vi "CSMinfo.vi"(4 "Error In":errorcluster, 7 "Command":string) -> (0 "Error Out":errorcluster, 3 "Response":string)   [LabVIEW 2018]
uses:
  MOKO_LabViewLibrary/MokoLowLevel/MokoLowLovelControl/MLLC_Mode.ctl
  data/CSMinfo.ctl
panel:
  in  "Utility name":string="CSMinfo"
  in  "Error Code":i32=5475
  in  "Settings":T2
  in  "Mode":T3=enum."Check"
  # "CSMinfo"
  # "Default Settings"
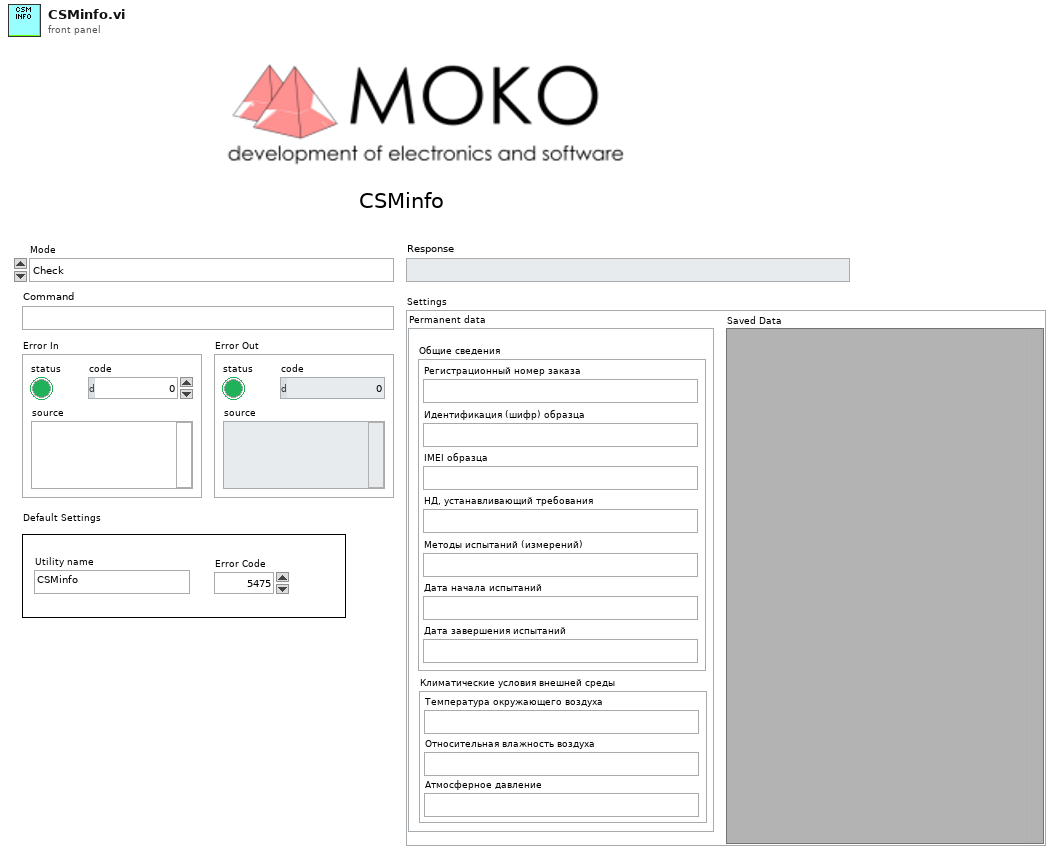
[diagram p1: front panel]
types:
  T1 = typedef "CSMinfo.ctl" = cluster{"Общие сведения":cluster{"Регистрационный номер заказа":string, "Идентификация (шифр) образца":string, "IMEI образца":string, "НД, устанавливающий требования":string, "Методы испытаний (измерений)":string, "Дата начала испытаний":string, "Дата завершения испытаний":string}, "Климатические условия внешней среды":cluster{"Температура окружающего воздуха":string, "Относительная влажность воздуха":string, "Атмосферное давление":string}}
  T2 = cluster{"Saved Data":variant, "Permanent data":T1}
  T3 = typedef "MLLC_Mode.ctl" = enum16{"get", "set", "close", "Init", "Check"}
  T4 = typedef "MLLC_Error.ctl" = errorcluster
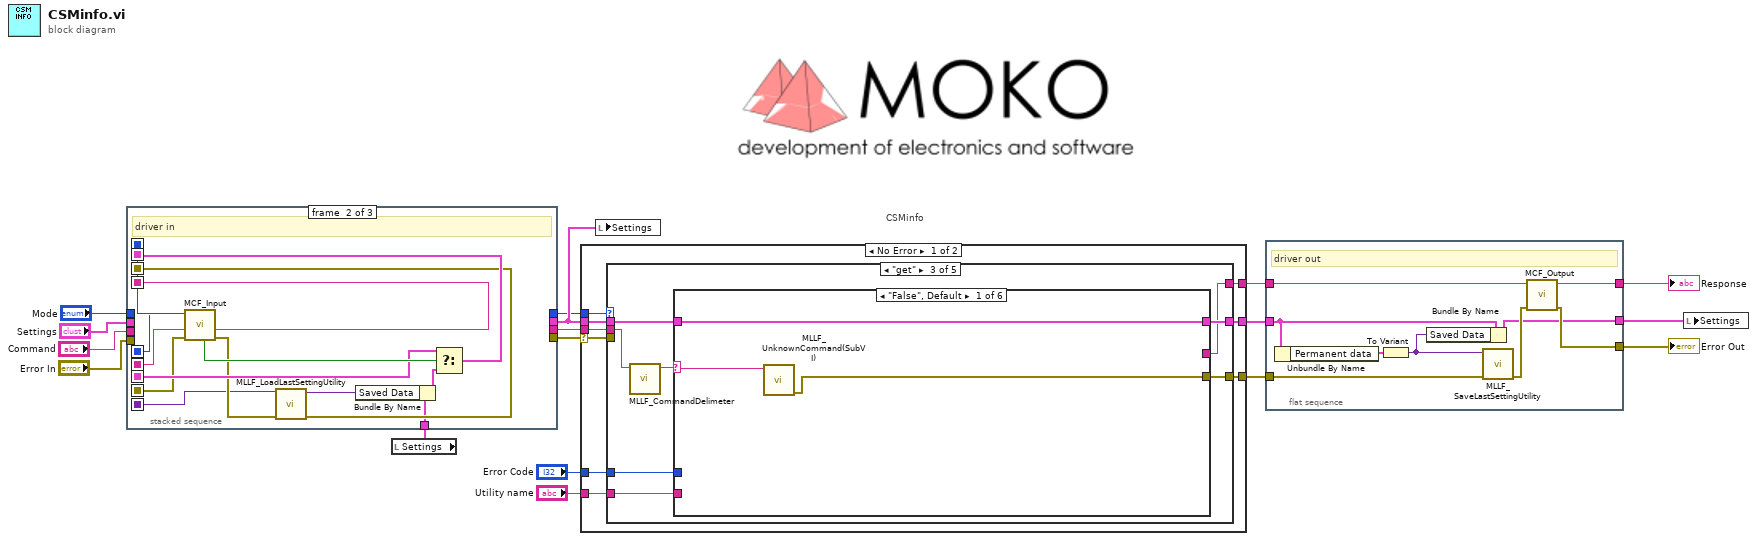
[diagram p0: block diagram]
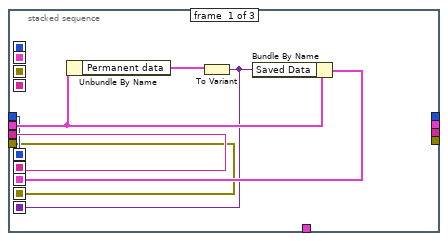
[diagram p2: hidden frame]
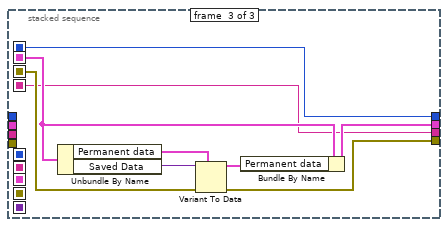
[diagram p3: hidden frame]
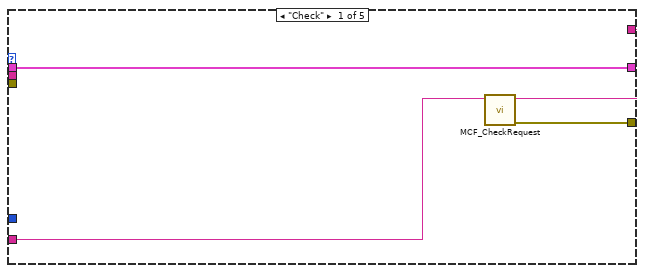
[diagram p4: hidden frame]
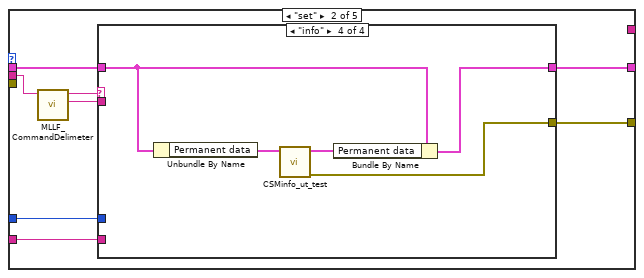
[diagram p5: hidden frame]
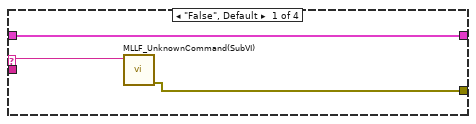
[diagram p6: hidden frame]
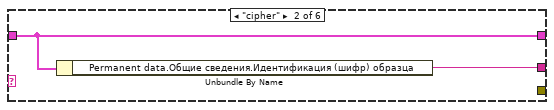
[diagram p9: hidden frame]
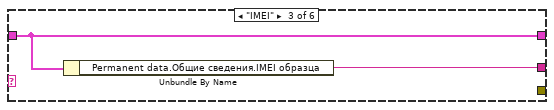
[diagram p10: hidden frame]
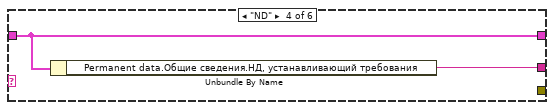
[diagram p11: hidden frame]
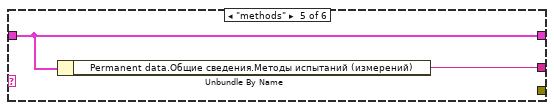
[diagram p12: hidden frame]
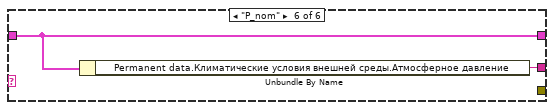
[diagram p13: hidden frame]
diagram:
  # "CSMinfo"
  n1 = local read "Settings"() -> (w12:T2)
  n2 = stacked-sequence {
    seq-local: [w20 _ _] -> [_ w36 _]
    seq-local: [w19 _ _] -> [_ w37 _]
    seq-local: [w22 _ _] -> [_ w32 _]
    seq-local: [w18 _ _] -> [_ w31 _]
    seq-local: [w21 _ _] -> [_ w26 _]
    seq-local: [_ w27 _] -> [_ _ w43]
    seq-local: [_ w38 _] -> [_ _ w40]
    seq-local: [_ w35 _] -> [_ _ w39]
    seq-local: [_ w34 _] -> [_ _ w44]
    tunnel: "Command" -> [w20 _ _]
    tunnel: "Mode" -> [w19 _ _]
    tunnel: "Error In" -> [w18 _ _]
    tunnel: "Settings" -> [w23 _ _]
    tunnel: w12 -> [_ w25 _]
    tunnel: [_ _ w39] -> w8
    tunnel: [_ _ w42] -> w11
    tunnel: [_ _ w41] -> w10
    tunnel: [_ _ w40] -> w9
    frame #0 {
      n3 = Unbundle By Name(w23) -> ("Permanent data"=w24:T1)
      n4 = To Variant(anything=w24) -> (Variant=w21:variant)
      n5 = Bundle By Name(cluster=w23, "Saved Data"=w21) -> (w22:T2)
    }
    frame #1 {
      # "driver in"
      n6 = call "MCF_Input.vi"("error in (no error)"=w31, "Command"=w36, "Mode"=w37) -> ("error out"=w30:errorcluster, "Command out"=w35:string, "Mode out"=w38:T3, "Boolean"=w33:bool)  [unwired: 5 in]
      n7 = call "MLLF_LoadLastSettingUtility.vi"("Error In"=w30, "Save data in"=w26) -> ("Error Out"=w27:errorcluster, "Save data out"=w29:variant)  [unwired: 8 in]
      n8 = Bundle By Name(cluster=w25, "Saved Data"=w29) -> (w28:T2)
      n9 = Select(t=w32, s=w33, f=w28) -> (s? t:f=w34:T2)
    }
    frame #2 {
      n10 = Unbundle By Name(w44) -> ("Permanent data"=w45:T1, "Saved Data"=w47:variant)
      n11 = Variant To Data(error in=w43, type=w45, Variant=w47) -> (data=w46:T1, error out=w41:errorcluster)
      n12 = Bundle By Name(cluster=w44, "Permanent data"=w46) -> (w42:T2)
    }
  }
  n13 = case shown="No Error" w10 {
    selector: w10 -> [w52 w103]
    tunnel: [w54 w103] -> w16
    tunnel: w9 -> [w56 _]
    tunnel: [w55 _] -> w14
    tunnel: w8 -> [w53 _]
    tunnel: w11 -> [w49 w102]
    tunnel: "Error Code" -> [w51 _]
    tunnel: "Utility name" -> [w50 _]
    tunnel: [w48 w102] -> w15
    frame No Error {
      n14 = case shown="\"get\"" w56 {
        tunnel: [w58 _ w80 _ _] -> w55
        tunnel: [w57 w67 w79 _ _] -> w54
        tunnel: w53 -> [_ w68 w86 _ _]
        tunnel: w52 -> [_ _ _ _ _]
        tunnel: w51 -> [_ w66 w84 _ _]
        tunnel: w50 -> [w59 w63 w83 _ _]
        tunnel: w49 -> [w60 w65 w85 w100 w101]
        tunnel: [w60 w64 w82 w100 w101] -> w48
        frame "Check" {
          n15 = call "MCF_CheckRequest.vi"("Driver Name"=w59) -> ("Error Out"=w57:errorcluster, "Output String"=w58:string)  [unwired: 9 in]
        }
        frame "set" {
          n16 = call "MLLF_CommandDelimeter.vi"("command with param"=w68) -> ("param 1"=w61:string, "command"=w62:string)  [unwired: 7 in, 2 out]
          n17 = case shown="\"info\"" w62 {
            selector: w62 -> [w70 _ _ _]
            tunnel: w61 -> [_ _ _ _]
            tunnel: [w69 _ _ w78] -> w67
            tunnel: w66 -> [_ _ _ _]
            tunnel: w65 -> [w71 w72 w73 w77]
            tunnel: [w71 w72 w73 w76] -> w64
            tunnel: w63 -> [_ _ _ _]
            frame "False", Default {
              n18 = call "MLLF_UnknownCommand(SubVI).vi"("Unknown command"=w70) -> ("error out"=w69:errorcluster)  [unwired: 10 in]
            }
            frame "<----MAIN FUNCTIONS---->" {
            }
            frame "---------ADDITIONAL---------" {
            }
            frame "info" {
              n19 = Unbundle By Name(w77) -> ("Permanent data"=w74:T1)
              n20 = call "CSMinfo_ut_test.vi"("CSMinfo in"=w74) -> ("Error Out"=w78:errorcluster, "CSMinfo out"=w75:T1)  [unwired: 9 in]
              n21 = Bundle By Name(cluster=w77, "Permanent data"=w75) -> (w76:T2)
            }
          }
        }
        frame "get" {
          n22 = call "MLLF_CommandDelimeter.vi"("command with param"=w86) -> ("command"=w81:string)  [unwired: 7 in, 3 out]
          n23 = case shown="\"False\", Default" w81 {
            selector: w81 -> [w88 _ _ _ _ _]
            tunnel: [w87 _ _ _ _ _] -> w79
            tunnel: w84 -> [_ _ _ _ _ _]
            tunnel: [w89 w90 w92 w94 w96 w98] -> w82
            tunnel: w85 -> [w89 w90 w92 w94 w96 w98]
            tunnel: w83 -> [_ _ _ _ _ _]
            tunnel: [_ w91 w93 w95 w97 w99] -> w80
            frame "False", Default {
              n24 = call "MLLF_UnknownCommand(SubVI).vi"("Unknown command"=w88) -> ("error out"=w87:errorcluster)  [unwired: 10 in]
            }
            frame "cipher" {
              n25 = Unbundle By Name(w90) -> ("Permanent data.Общие сведения.Идентификация (шифр) образца"=w91:string)
            }
            frame "IMEI" {
              n26 = Unbundle By Name(w92) -> ("Permanent data.Общие сведения.IMEI образца"=w93:string)
            }
            frame "ND" {
              n27 = Unbundle By Name(w94) -> ("Permanent data.Общие сведения.НД, устанавливающий требования"=w95:string)
            }
            frame "methods" {
              n28 = Unbundle By Name(w96) -> ("Permanent data.Общие сведения.Методы испытаний (измерений)"=w97:string)
            }
            frame "P_nom" {
              n29 = Unbundle By Name(w98) -> ("Permanent data.Климатические условия внешней среды.Атмосферное давление"=w99:string)
            }
          }
        }
        frame "close" {
        }
        frame "Init" {
        }
      }
    }
    frame Error {
    }
  }
  n30 = local write "Settings"(w11) -> ()
  n31 = flat-sequence {
    tunnel: [w112] -> w6
    tunnel: [w111] -> w4
    tunnel: w14 -> [w110]
    tunnel: w16 -> [w109]
    tunnel: w15 -> [w105]
    tunnel: [w107] -> w13
    frame #0 {
      # "driver out"
      n32 = Unbundle By Name(w105) -> ("Permanent data"=w104:T1)
      n33 = To Variant(anything=w104) -> (Variant=w106:variant)
      n34 = Bundle By Name(cluster=w105, "Saved Data"=w106) -> (w107:T2)
      n35 = call "MLLF_SaveLastSettingUtility.vi"("error in"=w109, "Saved Data"=w106) -> ("error out"=w108:T4)  [unwired: 8 in, 1 out]
      n36 = call "MCF_Output.vi"("Error In"=w108, "Input"=w110) -> ("Error Out"=w111:errorcluster, "Output"=w112:string)  [unwired: 8 in]
    }
  }
  n37 = local write "Settings"(w13) -> ()
  "Response" <- w6
  "Error Out" <- w4
